vi "空调监测配置同步 (子VI).vi"(11 "Boolean输入":refnum<vi>) -> ()   [LabVIEW 2016, in "环境动力监测库.lvlib" / "空调库.lvlib"]
uses:
  <vilib>/Utility/config.llb/NI_LVConfig.lvlib
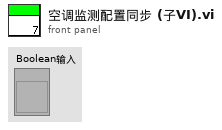
[diagram p1: front panel]
types:
  T1 = cluster{"分支":enum16{"open", "read", "write", "close"}, "字符串":string}
  T2 = cluster{"监测项描述:输出":string, "连接方式":enum16{"串口", "TCP"}, "端口":string, "IP address:":string, "Port:":string, "站号":u64, "传感器型号":string, "波特率":u64, "data bits":u64, "停止位":u16, "奇偶校验":u16}
  T3 = typedef "NI_LVConfig.lvlib/Config Data RefNum.ctl" = refnum<k1>
  T4 = cluster{"型号选择":enum16{"黑盾", "英维克", "仁科测控RS-KTC-N01"}, "MB session in":refnum<class "MB_Master.lvclass">, "英维克空调寄存器":u16[], "通讯状态":bool, "PORT":string, "IP":string, "Slave ID ":u8, "Serial Config":cluster{"baud rate (bps)":u32, "stop bits":u16, "parity":u16, "flow control":u16, "timeout":u32, "retries":i32}, "VISA Resource":refnum<visa-resource-name>, "MB通信方式选择":enum16{"串口", "TCP"}}
  T5 = cluster{"baud rate (bps)":u32, "stop bits":u16, "parity":u16, "flow control":u16, "timeout":u32, "retries":i32}
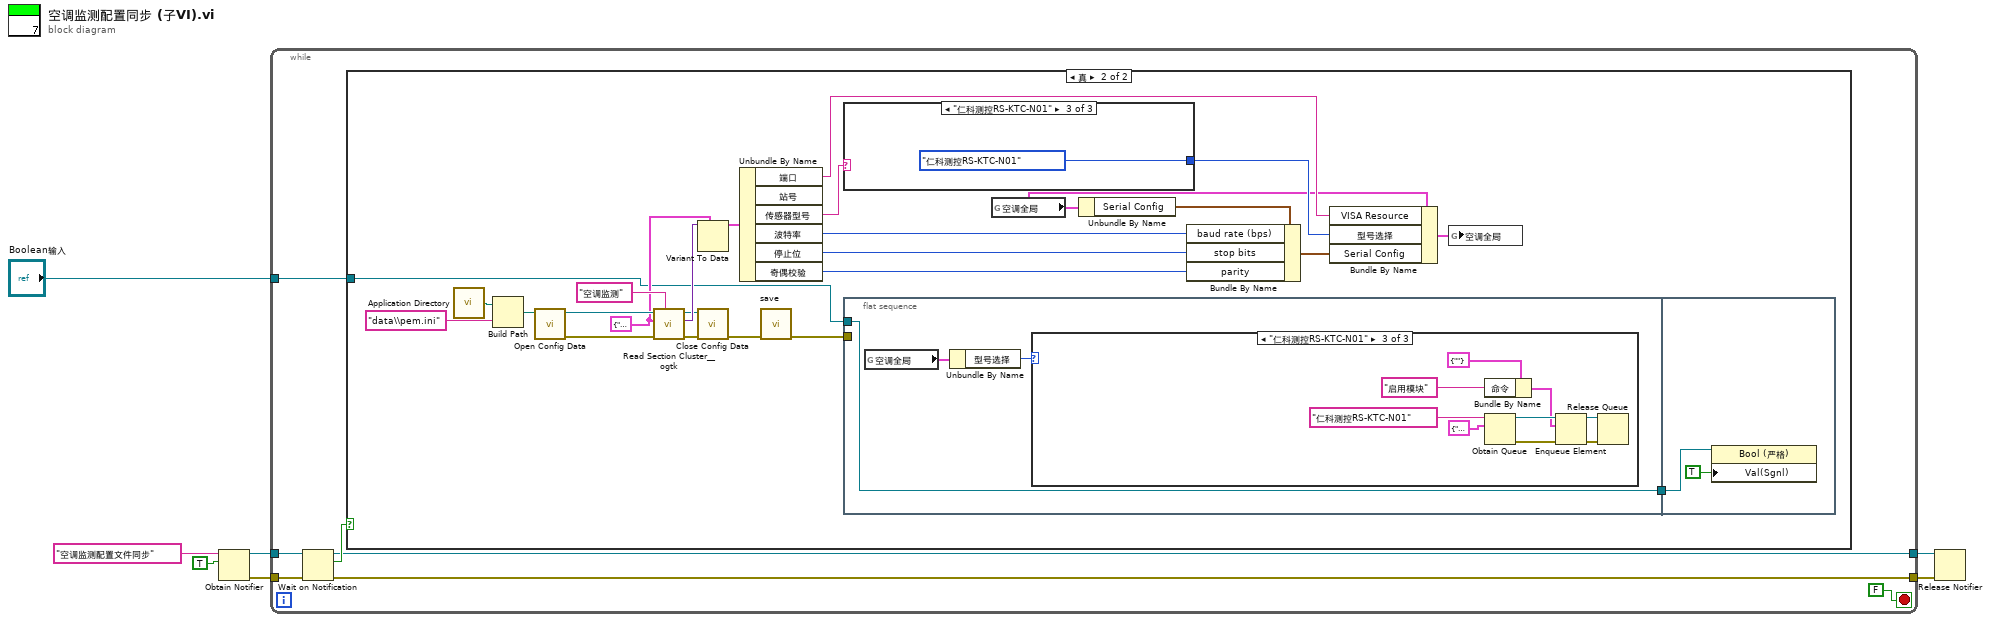
[diagram p0: block diagram]
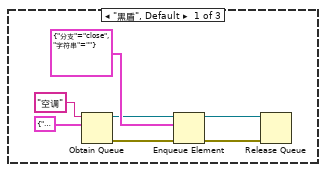
[diagram p3: hidden frame]
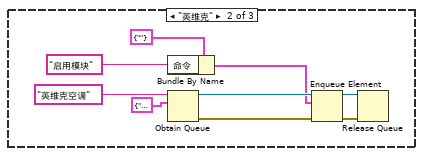
[diagram p4: hidden frame]
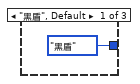
[diagram p5: hidden frame]
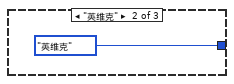
[diagram p6: hidden frame]
diagram:
  n1 = Obtain Notifier(name (unnamed)="空调监测配置文件同步" ("名称（未命名）"), notification data type=TRUE) -> (notifier out=w5:refnum<notifier>, error out=w4:errorcluster)  [unwired: 2 in, 1 out]
  n2 = while {
    tunnel: w5 -> [w14]
    tunnel: w4 -> [w13]
    tunnel: [w10] -> w3
    tunnel: [w9] -> w2
    tunnel: "Boolean输入" -> [w8]
    stop <- FALSE stop-if-true
    n3 = Wait on Notification(notifier=w14, error in (no error)=w13) -> (notifier out=w10:refnum<notifier>, notification=w12:bool, error out=w9:errorcluster)  [unwired: 2 in, 1 out]
    n4 = case shown="真" w12 {
      tunnel: w8 -> [_ w24]
      frame False {
      }
      frame True {
        w26 = T2 {"监测项描述:输出"="", "连接方式"=enum."串口", "端口"="", "IP address:"="", "Port:"="", "站号"=19200, "传感器型号"="", "波特率"=19200, "data bits"=8, "停止位"=10, "奇偶校验"=0} ("输入簇")
        n5 = call <vilib>:"Application Directory.vi"() -> ("Application Directory"=w30:path)
        n6 = Build Path(base path=w30, name or relative path="data\\pem.ini" ("名称或相对路径")) -> (appended path=w29:path)
        n7 = call <vilib>:"Open Config Data.vi"("configuration file path"=w29) -> ("error out"=w28:errorcluster, "refnum"=w27:T3)  [unwired: 8 in, 1 out]
        n8 = call <userlib>:"Read Section Cluster__ogtk.vi"("section (optional)"="空调监测", "error in (no error)"=w28, "Section Formatted Cluster Type"=w26, "refnum"=w27) -> ("error out"=w34:errorcluster, "Section Formatted Cluster"=w35:variant, "dup refnum"=w33:T3)  [unwired: 3 in, 2 out]
        n9 = Variant To Data(type=w26, Variant=w35) -> (data=w36:T2)  [unwired: 1 in, 1 out]
        n10 = call <vilib>:"Close Config Data.vi"("error in (no error)"=w34, "refnum"=w33) -> ("error out"=w22:errorcluster)  [unwired: 8 in, 1 out]
        n11 = Unbundle By Name(w36) -> ("端口"=w20:string, "传感器型号"=w25:string, "波特率"=w37:u64, "停止位"=w38:u16, "奇偶校验"=w39:u16)  [unwired: 1 out]
        n12 = call "save.vi"("error in (no error)"=w22) -> ("error out"=w21:errorcluster)  [unwired: 10 in]
        n13 = case shown="\"仁科测控RS-KTC-N01\"" w25 {
          tunnel: [enum16{"黑盾", "英维克", "仁科测控RS-KTC-N01"}."黑盾" ("型号选择") enum16{"黑盾", "英维克", "仁科测控RS-KTC-N01"}."英维克" ("型号选择") enum16{"黑盾", "英维克", "仁科测控RS-KTC-N01"}."仁科测控RS-KTC-N01" ("型号选择")] -> w19
          frame "黑盾", Default {
          }
          frame "英维克" {
          }
          frame "仁科测控RS-KTC-N01" {
          }
        }
        n14 = flat-sequence {
          tunnel: w24 -> [w42]
          tunnel: [w42] -> w23
          tunnel: w21 -> [_]
          tunnel: w23 -> [w68]
          frame #0 {
            n15 = global read "断电保存全局变量.vi" "空调全局"() -> (w41:T4)
            n16 = Unbundle By Name(w41) -> ("型号选择"=w40:enum16{"黑盾", "英维克", "仁科测控RS-KTC-N01"})
            n17 = case shown="\"仁科测控RS-KTC-N01\"" w40 {
              frame "黑盾", Default {
                n18 = Obtain Queue(name (unnamed)="空调" ("名称（未命名）"), element data type=T1 {"分支"=enum."open", "字符串"="获取系统模拟量量化数据"}) -> (queue out=w46:refnum<queue>, error out=w45:errorcluster)  [unwired: 3 in, 1 out]
                n19 = Enqueue Element(queue=w46, element=T1 {"分支"=enum."close", "字符串"=""} ("元素"), error in (no error)=w45) -> (queue out=w44:refnum<queue>, error out=w43:errorcluster)  [unwired: 1 in, 1 out]
                n20 = Release Queue(queue=w44, error in (no error)=w43) -> ()  [unwired: 1 in, 3 out]
              }
              frame "英维克" {
                n21 = Bundle By Name(cluster=cluster{"命令":string} {"命令"=""} ("元素"), "命令"="启用模块" ("名称（未命名）")) -> (w54:cluster{"命令":string})
                n22 = Obtain Queue(name (unnamed)="英维克空调" ("名称（未命名）"), element data type=cluster{"命令":string} {"命令"="启用模块"} ("元素")) -> (queue out=w57:refnum<queue>, error out=w58:errorcluster)  [unwired: 3 in, 1 out]
                n23 = Enqueue Element(queue=w57, element=w54, error in (no error)=w58) -> (queue out=w51:refnum<queue>, error out=w50:errorcluster)  [unwired: 1 in, 1 out]
                n24 = Release Queue(queue=w51, error in (no error)=w50) -> ()  [unwired: 1 in, 3 out]
              }
              frame "仁科测控RS-KTC-N01" {
                n25 = Bundle By Name(cluster=cluster{"命令":string} {"命令"=""} ("元素"), "命令"="启用模块" ("名称（未命名）")) -> (w63:cluster{"命令":string})
                n26 = Obtain Queue(name (unnamed)="仁科测控RS-KTC-N01" ("名称（未命名）"), element data type=cluster{"命令":string} {"命令"="启用模块"} ("元素")) -> (queue out=w66:refnum<queue>, error out=w67:errorcluster)  [unwired: 3 in, 1 out]
                n27 = Enqueue Element(queue=w66, element=w63, error in (no error)=w67) -> (queue out=w60:refnum<queue>, error out=w59:errorcluster)  [unwired: 1 in, 1 out]
                n28 = Release Queue(queue=w60, error in (no error)=w59) -> ()  [unwired: 1 in, 3 out]
              }
            }
          }
          frame #1 {
            n29 = property on="属性节点" class="Bool (严格)"(reference=w68, "Val(Sgnl)"=TRUE) -> ()  [unwired: 1 in, 2 out]
          }
        }
        n30 = global read "断电保存全局变量.vi" "空调全局"() -> (w17:T4)
        n31 = Unbundle By Name(w17) -> ("Serial Config"=w16:T5)
        n32 = Bundle By Name(cluster=w16, "baud rate (bps)"=w37, "stop bits"=w38, "parity"=w39) -> (w18:T5)
        n33 = Bundle By Name(cluster=w17, "VISA Resource"=w20, "型号选择"=w19, "Serial Config"=w18) -> (w15:T4)
        n34 = global write "断电保存全局变量.vi" "空调全局"(w15) -> ()
      }
    }
  }
  n35 = Release Notifier(notifier=w3, error in (no error)=w2) -> ()  [unwired: 1 in, 3 out]
